vi "CriticalLoadIndex.vi"() -> ()   [LabVIEW 2016]
panel:
  in  "Crit_Ind":i32[](array[numeric])
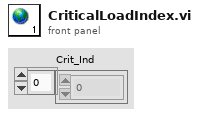
[diagram p1: front panel]
diagram:
